vi "PID Advanced Integral Action (DBL Array).vi"(0 "Ki":dbl[](array[numeric]) format="%.2f", 1 "proportional action":dbl[](array[numeric]) format="%.2f", 2 "error":dbl[](array[numeric]) format="%.2f", 3 "setpoint range":T1(array[cluster])=[{"setpoint high"=100.0, "setpoint low"=0.0}] {"setpoint high" format="%.2f"; "setpoint low" format="%.2f"}, 5 "PID gains":T2(array[cluster]) {"derivative time (Td, min)" format="%.3f"; "integral time (Ti, min)" format="%.3f"; "proportional gain (Kc)" format="%.3f"}, 7 "previous output":dbl[](array[numeric]) format="%.2f", 9 "derivative action":dbl[](array[numeric]) format="%.2f", 11 "initialize (F)":bool, 12 "dt (min)":dbl format="%.3f", 13 "output range":cluster{"output high":dbl, "output low":dbl}[](array[cluster]) {"output low" format="%.2f"; "output high" format="%.2f"}, 14 "auto? (T)":bool[](array[boolean])=[TRUE]) -> (6 "output":dbl[](array[numeric]) format="%.2f")   [LabVIEW 2020, in "NI_PID_pid.lvlib"]
uses:
  <vilib>/addons/control/pid/NI_PID_pid.lvlib
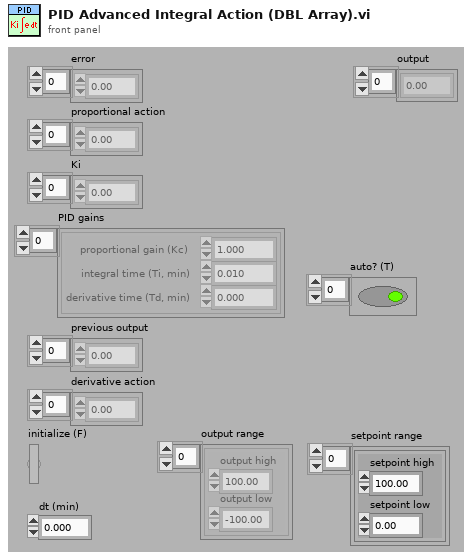
[diagram p1: front panel]
types:
  T1 = cluster{"setpoint high":dbl, "setpoint low":dbl}[]
  T2 = cluster{"proportional gain (Kc)":dbl, "integral time (Ti, min)":dbl, "derivative time (Td, min)":dbl}[]
  T3 = cluster{"proportional gain (Kc)":dbl, "integral time (Ti, min)":dbl, "derivative time (Td, min)":dbl}
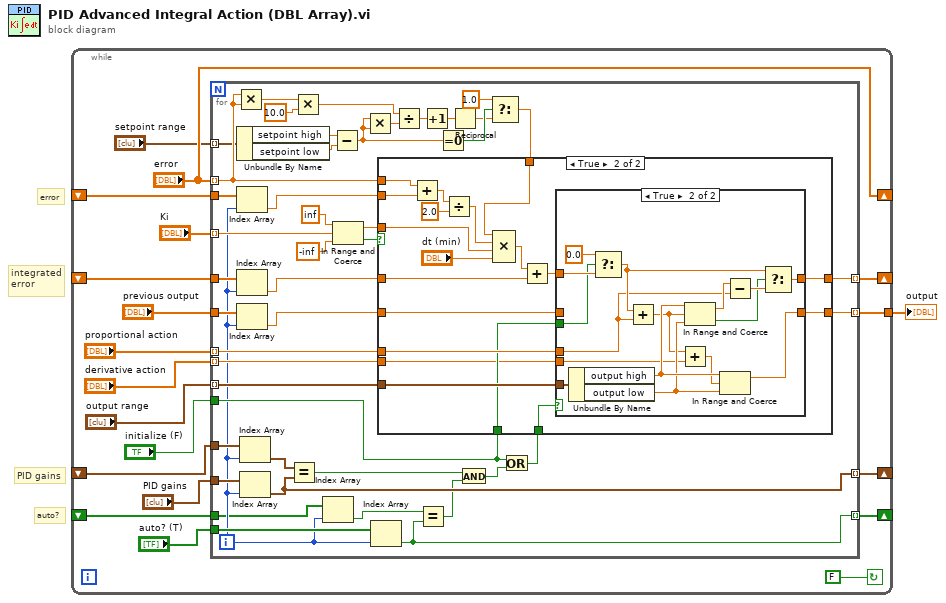
[diagram p0: block diagram]
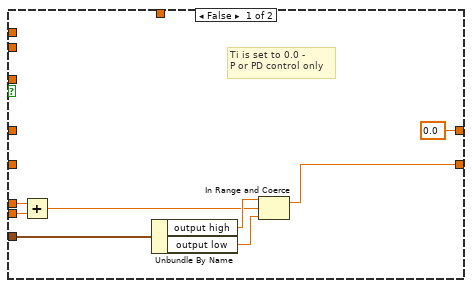
[diagram p2: hidden frame]
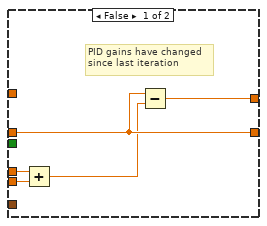
[diagram p3: hidden frame]
diagram:
  # "auto?"
  # "PID gains"
  # "integrated\nerror"
  # "error"
  n1 = while {
    tunnel: [w2] -> w1
    shift-left: _ -> [w8]
    shift-right: [w6] -> _
    shift-left: _ -> [w20]
    shift-right: ["error"] -> _
    shift-left: _ -> [w19]
    shift-right: [w18] -> _
    shift-left: _ -> [w9]
    shift-right: [w5] -> _
    stop <- FALSE continue-if-true
    n2 = for {
      tunnel: w20 -> [w32]
      tunnel: w19 -> [w30]
      tunnel: [w65] -> w18 mode=indexing
      tunnel: "proportional action" -> [w64] mode=indexing
      tunnel: "previous output" -> [w28]
      tunnel: [w60] -> w2 mode=indexing
      tunnel: "error" -> [w43] mode=indexing
      tunnel: "Ki" -> [w58] mode=indexing
      tunnel: "output range" -> [w57] mode=indexing
      tunnel: "setpoint range" -> [w42] mode=indexing
      tunnel: "derivative action" -> [w41] mode=indexing
      tunnel: "initialize (F)" -> [w26]
      tunnel: "PID gains" -> [w40]
      tunnel: w9 -> [w25]
      tunnel: w8 -> [w22]
      tunnel: "auto? (T)" -> [w39]
      tunnel: [w38] -> w6 mode=indexing
      tunnel: [w37] -> w5 mode=indexing
      i -> [w23]
      n3 = Multiply(x=w43, y=w43) -> (x*y=w50:dbl)
      n4 = Unbundle By Name(w42) -> ("setpoint high"=w56:dbl, "setpoint low"=w55:dbl)
      n5 = Index Array(array=w32, index=w23) -> (element=w31:dbl)
      n6 = Index Array(array=w30, index=w23) -> (element=w29:dbl)
      n7 = Index Array(array=w28, index=w23) -> (element=w27:dbl)
      n8 = Index Array(array=w25, index=w23) -> (element=w24:T3)
      n9 = Index Array(array=w40, index=w23) -> (element=w37:T3)
      n10 = Equal?(x=w24, y=w37) -> (x = y?=w34:bool)
      n11 = Multiply(x=w50, y=10.0) -> (x*y=w53:dbl)
      n12 = Index Array(array=w22, index=w23) -> (element=w21:bool)
      n13 = Subtract(x=w56, y=w55) -> (x-y=w48:dbl)
      n14 = In Range and Coerce(upper limit=inf, x=w58, lower limit=-inf) -> (coerced(x)=w59:dbl, In Range?=w61:bool)
      n15 = Multiply(x=w48, y=w48) -> (x*y=w49:dbl)
      n16 = Index Array(array=w39, index=w23) -> (element=w38:bool)
      n17 = Divide(x=w53, y=w49) -> (x/y=w52:dbl)
      n18 = Equal?(x=w21, y=w38) -> (x = y?=w33:bool)
      n19 = Increment(x=w52) -> (x+1=w51:dbl)
      n20 = Equal To 0?(x=w48) -> (x = 0?=w47:bool)
      n21 = Reciprocal(x=w51) -> (1/x=w46:dbl)
      n22 = And(x=w34, y=w33) -> (x .and. y?=w36:bool)
      n23 = Select(t=1.0, s=w47, f=w46) -> (s? t:f=w44:dbl)
      n24 = Or(x=w26, y=w36) -> (x .or. y?=w35:bool)
      n25 = case shown="True" w61 {
        tunnel: w43 -> [_ w91]
        tunnel: w31 -> [_ w92]
        tunnel: w29 -> [_ w86]
        tunnel: [0.0 ("t") w81] -> w65
        tunnel: w59 -> [_ w79]
        tunnel: w64 -> [w67 w84]
        tunnel: [w73 w80] -> w60
        tunnel: w57 -> [w72 w82]
        tunnel: w27 -> [_ w83]
        tunnel: w26 -> [_ w77]
        tunnel: w35 -> [_ w76]
        tunnel: w44 -> [_ w75]
        tunnel: w41 -> [w68 w74]
        frame False {
          # "Ti is set to 0.0 -\nP or PD control only"
          n26 = Add(x=w67, y=w68) -> (x+y=w66:dbl)
          n27 = Unbundle By Name(w72) -> ("output high"=w71:dbl, "output low"=w70:dbl)
          n28 = In Range and Coerce(upper limit=w71, x=w66, lower limit=w70) -> (coerced(x)=w73:dbl)  [unwired: 1 out]
        }
        frame True {
          n29 = Add(x=w91, y=w92) -> (x+y=w89:dbl)
          n30 = Divide(x=w89, y=2.0) -> (x/y=w88:dbl)
          n31 = Compound Arithmetic op=MULTIPLY(w75, w88, w79, "dt (min)") -> (w87:dbl)
          n32 = Add(x=w87, y=w86) -> (x+y=w85:dbl)
          n33 = case shown="True" w76 {
            tunnel: w85 -> [_ w104]
            tunnel: w84 -> [w94 w102]
            tunnel: w83 -> [w97 _]
            tunnel: w77 -> [_ w103]
            tunnel: w82 -> [_ w101]
            tunnel: [w96 w99] -> w81
            tunnel: [w97 w100] -> w80
            tunnel: w74 -> [w95 w98]
            frame False {
              # "PID gains have changed\nsince last iteration"
              n34 = Add(x=w94, y=w95) -> (x+y=w93:dbl)
              n35 = Subtract(x=w97, y=w93) -> (x-y=w96:dbl)
            }
            frame True {
              n36 = Unbundle By Name(w101) -> ("output high"=w111:dbl, "output low"=w110:dbl)
              n37 = Select(t=0.0, s=w103, f=w104) -> (s? t:f=w107:dbl)
              n38 = Add(x=w107, y=w102) -> (x+y=w106:dbl)
              n39 = Add(x=w106, y=w98) -> (x+y=w105:dbl)
              n40 = In Range and Coerce(upper limit=w111, x=w106, lower limit=w110) -> (coerced(x)=w109:dbl, In Range?=w108:bool)
              n41 = In Range and Coerce(upper limit=w111, x=w105, lower limit=w110) -> (coerced(x)=w100:dbl)  [unwired: 1 out]
              n42 = Subtract(x=w109, y=w102) -> (x-y=w112:dbl)
              n43 = Select(t=w107, s=w108, f=w112) -> (s? t:f=w99:dbl)
            }
          }
        }
      }
    }
  }
  "output" <- w1
